vi "FRP_Query.vi"(0 "System no.":i32=1 min=1 max=4 step=1, 2 "Routines to query":string[](array[string]), 3 "All routines?":bool, 5 "error in":errorcluster) -> (14 "Status":i32[](array[numeric]), 19 "error out":errorcluster)   [LabVIEW 2020]
doc: "Returns current status of given fast alignment routine(s). \n\nC-887, E-727.AS: Status can be\n0 - given routinehas been stopped / is not running\n2 - given routineis running\n\nE-712: Status can be\n0 - given routinehas been stopped / is not running\n1 - given routinehas been paused\n2 - given routineis running\n\nC-887, E-712, E-727.AS:"
panel:
  # "Returns current status of given fast alignment procedure(s)."
  # "Query"
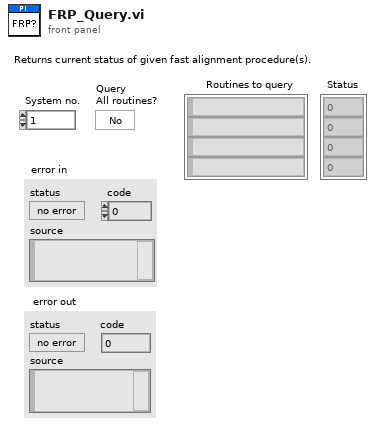
[diagram p1: front panel]
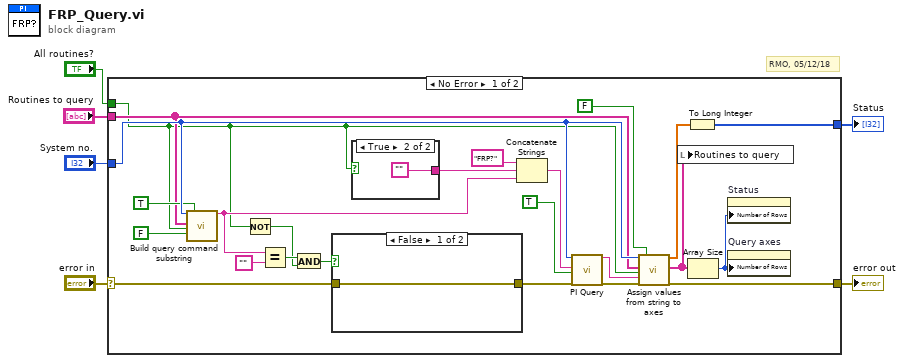
[diagram p0: block diagram]
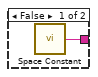
[diagram p2: hidden frame]
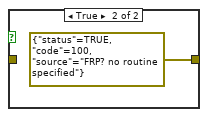
[diagram p3: hidden frame]
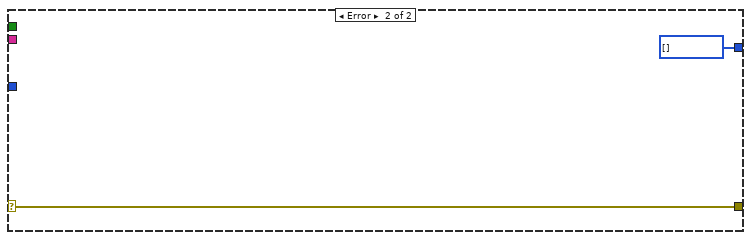
[diagram p4: hidden frame]
diagram:
  # "RMO, 05/12/18"
  n1 = case shown="No Error" "error in" {
    selector: "error in" -> [w7 w35]
    tunnel: [w16 i32[] [] ("Values")] -> w6
    tunnel: "Routines to query" -> [w13 _]
    tunnel: [w14 w35] -> w4
    tunnel: "System no." -> [w22 _]
    tunnel: "All routines?" -> [w12 _]
    frame No Error {
      n2 = call "Build query command substring.vi"("System no."=w22, "Axes to query in"=w13, "Query\nAll axes?"=w12, "For all axes: use\nAxis identifier?"=FALSE ("For all axes: use\nAxis identifier?"), "With space?"=TRUE) -> ("Command substring"=w25:string)  [unwired: 1 in, 13 out]
      n3 = Not(x=w12) -> (.not. x?=w23:bool)
      n4 = Equal?(x=w25, y="" ("x")) -> (x = y?=w24:bool)
      n5 = And(x=w24, y=w23) -> (x .and. y?=w26:bool)
      n6 = case shown="False" w26 {
        tunnel: [w33 errorcluster {"status"=TRUE, "code"=100, "source"="FRP? no routine specified"} ("error out")] -> w15
        tunnel: w7 -> [w33 _]
        frame False {
        }
        frame True {
        }
      }
      n7 = case shown="True" w12 {
        tunnel: [w31 ""] -> w10
        frame False {
          n8 = call "Space Constant.vi"() -> ("String"=w31:string)
        }
        frame True {
        }
      }
      n9 = Concatenate Strings("FRP?", w10, w25) -> (w29:string)
      n10 = call "PI Query.vi"("System no."=w22, "String to send"=w29, "Attach termination char.?"=TRUE ("Attach Linefeed?"), "error in"=w15) -> ("String read"=w9:string, "error out"=w8:errorcluster)  [unwired: 3 in, 11 out]
      n11 = call "Assign values from string to axes.vi"("System no."=w22, "Queried axes"=w13, "All axes queried?"=w12, "Input String"=w9, "error in"=w8, "Axes related?"=FALSE) -> ("Values"=w28:dbl[], "Queried axes out"=w17:string[], "error out"=w14:errorcluster)  [unwired: 3 in, 8 out]
      n12 = local write "Routines to query"(w17) -> ()
      n13 = To Long Integer(number=w28) -> (32bit integer=w16:i32[])
      n14 = Array Size(array=w17) -> (size(s)=w18:i32)
      n15 = property on="Status" class="Arr (strict)"("Number of Rows"=w18) -> ()  [unwired: 2 in, 2 out]
      n16 = property on="Query axes" class="Arr (strict)"("Number of Rows"=w18) -> ()  [unwired: 2 in, 2 out]
    }
    frame Error {
    }
  }
  "error out" <- w4
  "Status" <- w6
